vi "Read Test Data (Manual Mode).vi"(0 "VISA resource name":refnum<visa-resource-name>, 11 "error in (no error)":errorcluster) -> (4 "VISA resource name out":refnum<visa-resource-name>, 6 "Test Meter Data Output":T1 {"Frequency (Hz)" format="%.1f"; "Voltage (V)" format="%.1f"; "RMS Current (A)" format="%.3f"; "Power (W)" format="%.1f"; "Peak Current (A)" format="%.1f"; "Power Factor" format="%.3f"; "Timer (s)" format="%.1f"}, 15 "error out":errorcluster)   [LabVIEW 2020, in "eec 6700.lvlib"]
doc: "Reads the Manual mode <B>active data being displayed on the LCD display</B> while the test is in process. It also gives the last data taken when the test sequence compled. \n\nIn Manual Mode the output data cluster has the following data.\n\n1. Memory\n2. Timer (s) - Not Supported in Firmware Version2.0\n3. Frequency (Hz)\n4. Voltage (V)\n5. RMS Current (A)\n6. Peak Current (A)\n7. Power (W)\n8. Power Factor\n9. Status"
uses:
  <instrlib>/eec 6700/eec 6700.lvlib
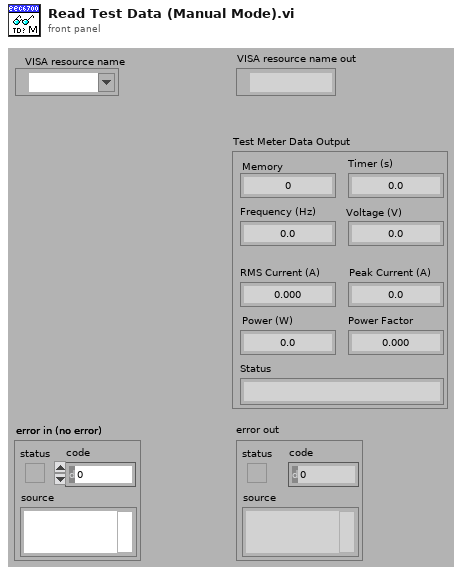
[diagram p1: front panel]
types:
  T1 = cluster{"Memory":dbl, "Timer (s)":dbl, "Frequency (Hz)":dbl, "Voltage (V)":dbl, "RMS Current (A)":dbl, "Peak Current (A)":dbl, "Power (W)":dbl, "Power Factor":dbl, "Status":string}
  T2 = cluster{"Memory":i32, "Timer":dbl, "Frequency":dbl, "Volt":dbl, "Current":dbl, "Peak Current":dbl, "Power":dbl, "Power Factor":dbl, "Status":string}
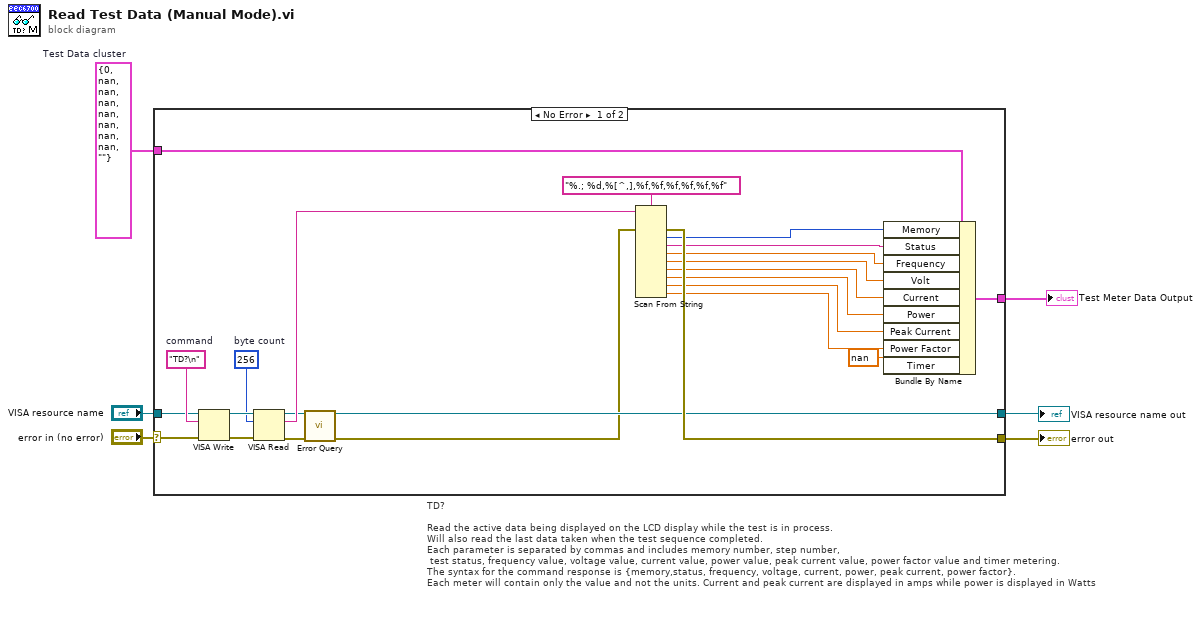
[diagram p0: block diagram]
diagram:
  w2 = T2 {"Memory"=0, "Timer"=nan, "Frequency"=nan, "Volt"=nan, "Current"=nan, "Peak Current"=nan, "Power"=nan, "Power Factor"=nan, "Status"=""}  # Test Data cluster
  # "TD?\n\nRead the active data being displayed on the LCD display while the test is in process. \nWill also read the last data taken when the test sequence completed. \nEach parameter is separated by commas and includes memory number, step number,\n test status, frequency value, voltage value, current value, power value, peak current value, power factor value and timer metering. \nThe syntax for the command response is {memory,status, frequency, voltage, current, power, peak current, power factor}. \nEach meter will contain only the value and not the units. Current and peak current are displayed in amps while power is displayed in Watts"
  n1 = case shown="No Error" "error in (no error)" {
    selector: "error in (no error)" -> [w23 w32]
    tunnel: "VISA resource name" -> [w24 w33]
    tunnel: [w8 w33] -> w4
    tunnel: [w22 w32] -> w3
    tunnel: [w27 w31] -> w1
    tunnel: w2 -> [w26 w31]
    frame No Error {
      w25 = "TD?\n"  # command
      w28 = u32 256  # byte count
      n2 = VISA Write(VISA resource name=w24, write buffer=w25, error in (no error)=w23) -> (VISA resource name out=w30:refnum<visa-resource-name>, error out=w29:errorcluster)  [unwired: 1 out]
      n3 = VISA Read(VISA resource name=w30, byte count=w28, error in (no error)=w29) -> (VISA resource name out=w20:refnum<visa-resource-name>, read buffer=w21:string, error out=w19:errorcluster)  [unwired: 1 out]
      n4 = call <instrlib>:"Error Query.vi"("VISA resource name"=w20, "error in (no error)"=w19) -> ("VISA resource name out"=w8:refnum<visa-resource-name>, "error out"=w7:errorcluster)  [unwired: 10 in, 2 out]
      n5 = Scan From String(format string="%.; %d,%[^,],%f,%f,%f,%f,%f,%f", input string=w21, error in=w7) -> (error out=w22:errorcluster, output 1=w17:i32, output 2=w16:string, output 3=w15:dbl, output 4=w14:dbl, output 5=w13:dbl, output 6=w12:dbl, output 7=w11:dbl, output 8=w10:dbl)  [unwired: 9 in, 2 out]
      n6 = Bundle By Name(cluster=w26, "Memory"=w17, "Status"=w16, "Frequency"=w15, "Volt"=w14, "Current"=w13, "Power"=w12, "Peak Current"=w11, "Power Factor"=w10, "Timer"=nan) -> (w27:T2)
    }
    frame Error {
    }
  }
  "VISA resource name out" <- w4
  "error out" <- w3
  "Test Meter Data Output" <- w1
